vi "read_rn16_v1.vi"() -> ()   [LabVIEW 2015]
panel:
  out "Numeric":i32
  out "Array 2":dbl[](array[numeric])
  out "Array":dbl[](array[numeric])
  out "Signals":dynamicdata(graph)
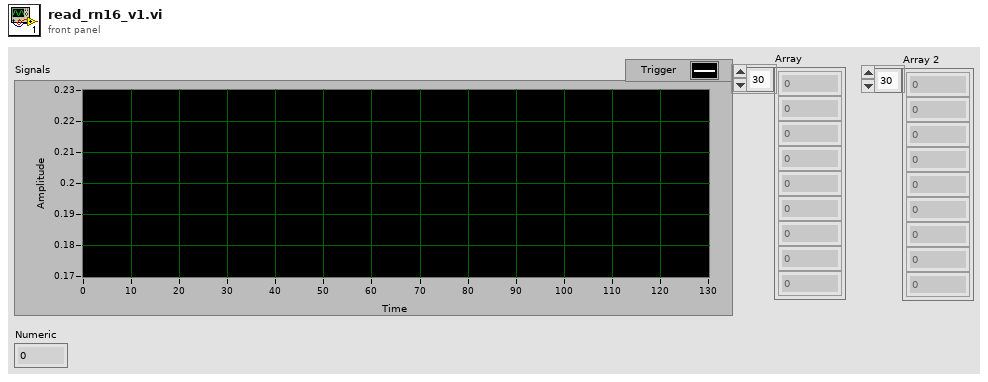
[diagram p1: front panel]
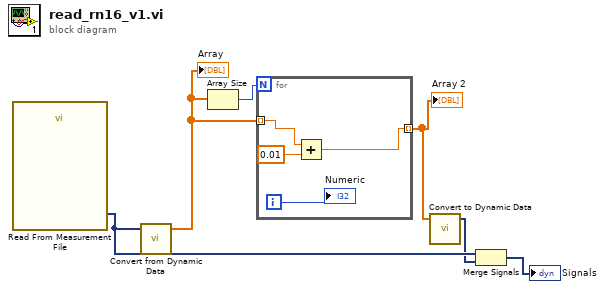
[diagram p0: block diagram]
diagram:
  n1 = call "Read From Measurement File"() -> ("Signals"=w6:dynamicdata)  [unwired: 6 in, 5 out]
  n2 = call "Convert from Dynamic Data"("Dynamic Data Type"=w6) -> ("Array"=w4:dbl[])  [unwired: 3 in]
  "Array" <- w4
  n3 = Array Size(array=w4) -> (size(s)=w5:i32)
  n4 = for {
    N: w5 -> [_]
    tunnel: w4 -> [w10] mode=indexing
    tunnel: [w8] -> w3 mode=indexing
    i -> [w7]
    n5 = Add(x=w10, y=0.01) -> (x+y=w8:dbl)
    "Numeric" <- w7
  }
  "Array 2" <- w3
  n6 = call "Convert to Dynamic Data"("Array"=w3) -> ("Dynamic Data Type"=w1:dynamicdata)  [unwired: 3 in]
  n7 = Merge Signals(w6, w1) -> (→"Signals":dynamicdata)
